vi "ControlSolenoids.vi"(0 "Joystick Refnum Name":string) -> ()   [LabVIEW 2014]
uses:
  <vilib>/Rock Robotics/WPI/Joystick/WPI_JoystickGetSetRefNum.vi
  <vilib>/Rock Robotics/WPI/Solenoid/WPI_SolenoidSetEnum.vi
  <vilib>/Rock Robotics/Network Tables/SD Write Boolean Array.vi
  <vilib>/Rock Robotics/Network Tables/SD Write Numeric Array.vi
  Robot Global Data.vi
  <vilib>/Rock Robotics/WPI/Solenoid/WPI_SolenoidGetEnum.vi
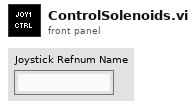
[diagram p1: front panel]
types:
  T1 = typedef "WPI_JoystickDevRef.ctl" = cluster{"Device":T2}
  T2 = typedef "WPI_JoystickDeviceEnum.ctl" = enum16{"USB 0", "USB 1", "USB 2", "USB 3", "USB 4", "USB 5"}
  T3 = typedef "WPI_SolenoidDevRef.ctl" = cluster{"DevStatus":errorcluster, "Pneumatics Control Module":u8, "Forward Solenoid Channel":T4, "Reverse Solenoid Channel":T4}
  T4 = typedef "WPI_SolenoidChannel.ctl" = enum8{"Solenoid 0", "Solenoid 1", "Solenoid 2", "Solenoid 3", "Solenoid 4", "Solenoid 5", "Solenoid 6", "Solenoid 7", "Invalid"}
  T5 = typedef "WPI_SolenoidValue.ctl" = enum16{"Off", "On", "Forward", "Reverse"}
  T6 = typedef "WPI_MotorControlDeviceRef.ctl" = cluster{"DeviceStatus":errorcluster, "Type":T7, "PWM":cluster{"Controller":T8, "PWM Channel":T9, "DeadBand":T10}, "CAN":cluster{"Device Number":u8, "Control Mode":T11, "Semaphore":T12, "Max Vout":dbl, "TalonSRX Control Mode":T13}, "Invert":bool, "TransformRef":T14, "InvTransformRef":T14}
  T7 = typedef "WPI_MotorControlType.ctl" = enum16{"PWM", "CAN", "CANTalonSRX"}
  T8 = typedef "FPGA_TypedefDigitalModule.ctl" = enum16{"Controller 1"}
  T9 = typedef "FPGA_DIOPWMChannel.ctl" = enum8{"PWM 0", "PWM 1", "PWM 2", "PWM 3", "PWM 4", "PWM 5", "PWM 6", "PWM 7", "PWM 8", "PWM 9", "PWM MXP 0", "PWM MXP 1", "PWM MXP 2", "PWM MXP 3", "PWM MXP 4", "PWM MXP 5", "PWM MXP 6", "PWM MXP 7", "PWM MXP 8", "PWM MXP 9", "Invalid"}
  T10 = typedef "WPI_PWMDeadband.ctl" = cluster{"Name":string, "maxPositivePwm":i32, "minPositivePwm":i32, "centerPwm":i32, "maxNegativePwm":i32, "minNegativePwm":i32, "angularRange":u16}
  T11 = typedef "WPI_CANJaguar_ControlMode.ctl" = enum8{"Percent VBus", "Current", "Speed", "Position", "Voltage"}
  T12 = typedef "Semaphore RefNum" = refnum<k1>
  T13 = typedef "WPI_CANTalonSRX_APIControlMode.ctl" = enum8{"Percent VBus", "Speed", "Position", "Slave", "Unchanged / Invalid"}
  T14 = typedef "WPI_PWMTransform_ConPane.ctl" = refnum<vi>
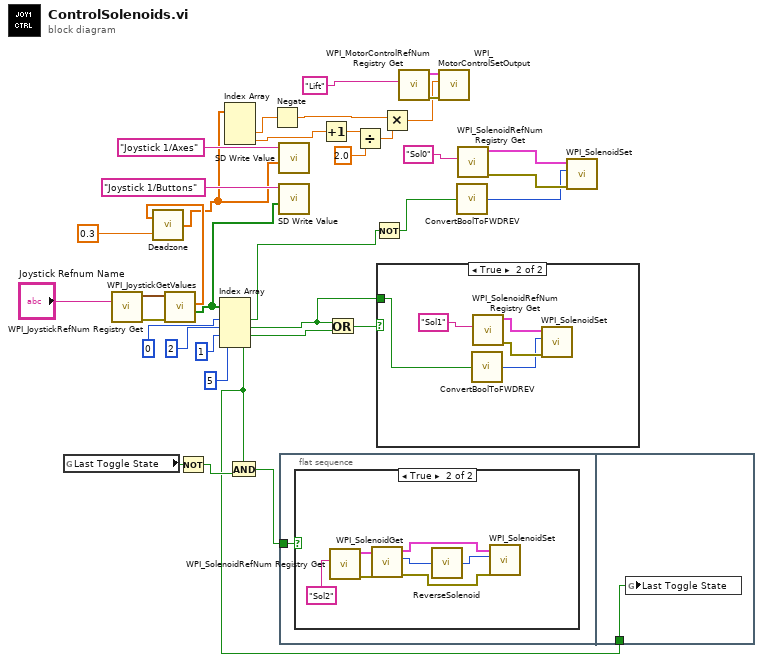
[diagram p0: block diagram]
diagram:
  n1 = global read "Robot Global Data.vi" "Last Toggle State"() -> (w20:bool)
  n2 = call <vilib>:"WPI_JoystickRefNum Registry Get.vi"("refnum name"="Joystick Refnum Name") -> ("error out"=w35:errorcluster, "JoystickDevRef"=w34:T1)  [unwired: 9 in]
  n3 = call <vilib>:"WPI_JoystickGetValues.vi"("error in (no error)"=w35, "JoystickDevRef"=w34) -> ("Buttons"=w14:bool[], "Axes"=w9:dbl[])  [unwired: 5 in, 3 out]
  n4 = call "Deadzone.vi"("Deadzone"=0.3, "Joystick Axes In"=w9) -> ("Joystick Axes Out"=w8:dbl[])
  n5 = Not(x=w20) -> (.not. x?=w19:bool)
  n6 = Index Array(array=w14, index #1=0, index #2=2, index #3=1, index #4=5) -> (element #1=w25:bool, element #2=w21:bool, element #3=w23:bool, element #4=w17:bool)
  n7 = Index Array(array=w8) -> (element #2=w7:dbl, element #3=w6:dbl)  [unwired: 3 in, 1 out]
  n8 = And(x=w17, y=w19) -> (x .and. y?=w18:bool)
  n9 = Negate(x=w7) -> (-x=w2:dbl)
  n10 = call-poly <vilib>:"SD Write Value.vi"("Numeric Array"=w8, "Name"="Joystick 1/Axes") -> ()  [unwired: 8 in, 2 out]
  n11 = call-poly <vilib>:"SD Write Value.vi"("Boolean Array"=w14, "Name"="Joystick 1/Buttons") -> ()  [unwired: 8 in, 2 out]
  n12 = flat-sequence {
    tunnel: w18 -> [w37]
    tunnel: w17 -> [w45]
    frame #0 {
      n13 = case shown="True" w37 {
        frame False {
        }
        frame True {
          n14 = call <vilib>:"WPI_SolenoidRefNum Registry Get.vi"("refnum name"="Sol2") -> ("error out"=w43:errorcluster, "SolenoidDevRef"=w42:T3)  [unwired: 9 in]
          n15 = call-poly <vilib>:"WPI_SolenoidGet.vi"("error in (no error)"=w43, "SolenoidDevRef"=w42) -> ("error out"=w39:errorcluster, "Value"=w41:T5, "SolenoidDevRef"=w38:T3)  [unwired: 7 in]
          n16 = call "ReverseSolenoid.vi"("Value In"=w41) -> ("Value Out"=w40:u8)
          n17 = call-poly <vilib>:"WPI_SolenoidSet.vi"("error in (no error)"=w39, "Value"=w40, "SolenoidDevRef"=w38) -> ()  [unwired: 7 in, 2 out]
        }
      }
    }
    frame #1 {
      n18 = global write "Robot Global Data.vi" "Last Toggle State"(w45) -> ()
    }
  }
  n19 = Increment(x=w6) -> (x+1=w5:dbl)
  n20 = Or(x=w21, y=w23) -> (x .or. y?=w22:bool)
  n21 = Divide(x=w5, y=2.0) -> (x/y=w3:dbl)
  n22 = Not(x=w25) -> (.not. x?=w24:bool)
  n23 = case shown="True" w22 {
    tunnel: w21 -> [_ w46]
    frame False {
    }
    frame True {
      n24 = call "ConvertBoolToFWDREV.vi"("Bool In"=w46) -> ("Direction Out"=w47:u8)
      n25 = call <vilib>:"WPI_SolenoidRefNum Registry Get.vi"("refnum name"="Sol1") -> ("error out"=w49:errorcluster, "SolenoidDevRef"=w48:T3)  [unwired: 9 in]
      n26 = call-poly <vilib>:"WPI_SolenoidSet.vi"("error in (no error)"=w49, "Value"=w47, "SolenoidDevRef"=w48) -> ()  [unwired: 7 in, 2 out]
    }
  }
  n27 = Multiply(x=w2, y=w3) -> (x*y=w1:dbl)
  n28 = call <vilib>:"WPI_MotorControlRefNum Registry Get.vi"("refnum name"="Lift") -> ("error out"=w12:errorcluster, "MotorControlDevRef"=w11:T6)  [unwired: 9 in]
  n29 = call <vilib>:"WPI_MotorControlSetOutput.vi"("error in (no error)"=w12, "Output"=w1, "MotorControlDevRef"=w11) -> ()  [unwired: 6 in, 3 out]
  n30 = call "ConvertBoolToFWDREV.vi"("Bool In"=w24) -> ("Direction Out"=w26:u8)
  n31 = call <vilib>:"WPI_SolenoidRefNum Registry Get.vi"("refnum name"="Sol0") -> ("error out"=w28:errorcluster, "SolenoidDevRef"=w27:T3)  [unwired: 9 in]
  n32 = call-poly <vilib>:"WPI_SolenoidSet.vi"("error in (no error)"=w28, "Value"=w26, "SolenoidDevRef"=w27) -> ()  [unwired: 7 in, 2 out]
